vi "FTW-ScripterStep-Base_StartTime.vi"(0 "FTW-ScripterStep-Base in":refnum<class "FTW-ScripterStep-Base.lvclass">, 11 "error in (no error)":errorcluster) -> (4 "FTW-ScripterStep-Base out":refnum<class "FTW-ScripterStep-Base.lvclass">, 15 "error out":errorcluster)   [LabVIEW 2015, in "FTW-ScripterStep-Base.lvclass"]
uses:
  FTW-ScripterStep-Base.lvclass
  FTW-ScripterStep-Base.lvclass/FTW-ScripterStep-Base.ctl
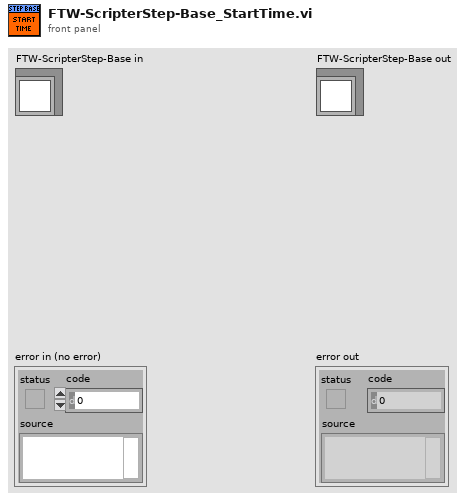
[diagram p1: front panel]
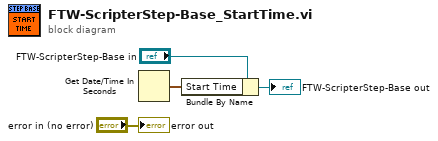
[diagram p0: block diagram]
diagram:
  n1 = Get Date/Time In Seconds() -> (seconds since 1Jan1904=w1:timestamp)
  n2 = Bundle By Name(cluster="FTW-ScripterStep-Base in", "Start Time"=w1) -> (→"FTW-ScripterStep-Base out":refnum<class "FTW-ScripterStep-Base.lvclass">)
  "error out" <- "error in (no error)"
